vi "sample rack.vi"(0 "Sample Tray":T2, 1 "vial status":enum16{"Empty", "Filling", "Full"}[](array[ring]), 2 "colors":u32[](array[colorbox])=[61185, 16383786, 2621695], 4 "Gilson ID":i32) -> (3 "scale":dbl[unit], 5 "vial position":T5, 6 "Sample Tray out":T2)   [LabVIEW 2012]
uses:
  point.ctl
  file action.ctl
  vial position.ctl
  toolbar icons/Save calibration.ctl
  toolbar icons/Open calibration.ctl
panel:
  out "Coords":cluster{"Horizontal":i32, "Vertical":i32}
  out "Array":bool[](array[boolean])
  out "vial radius":dbl
  out "vial graph centers":cluster{"x":dbl, "y":dbl}[](array[cluster])
  in  "Open sample tray":T3
  in  "Save sample tray":T4
  in  "OK Button":bool
  in  "Model 222 range":T1={"x"=0.39299999999999996, "y"=0.244}
  out "sample tray":picture
  # "Click on vial to move sample changer to that position"
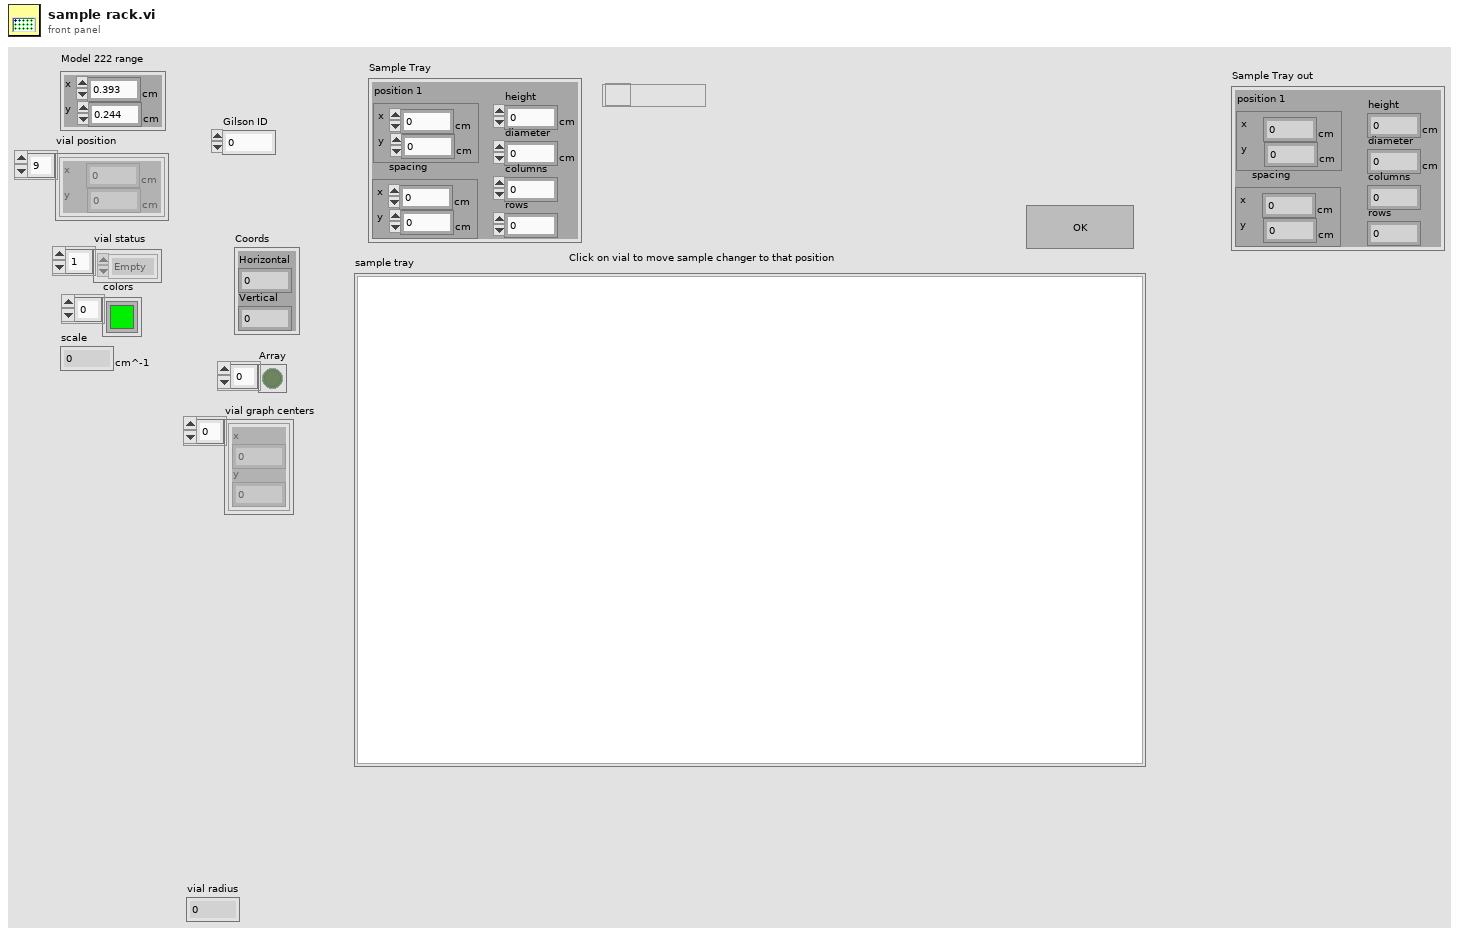
[diagram p1: front panel]
types:
  T1 = typedef "point.ctl" = cluster{"x":dbl[unit], "y":dbl[unit]}
  T2 = cluster{"diameter":dbl[unit], "height":dbl[unit], "columns":u16, "rows":u16, "position 1":T1, "spacing":T1}
  T3 = typedef "Open calibration.ctl" = bool
  T4 = typedef "Save calibration.ctl" = bool
  T5 = typedef "vial position.ctl" = T1[]
  T6 = cluster{"Width":u16, "Style":enum32{"Solid", "Dash", "Dot", "DashDot", "DashDotDot"}}
  T7 = typedef "file action.ctl" = enum16{"Save", "Open"}
  T8 = typedef "LVBoundsTypeDef.ctl" = cluster{"Width":u32, "Height":u32}
  T9 = typedef "LVMouseTypeDef.ctl" = cluster{"Mouse Position":cluster{"X":i32, "Y":i32}, "Mouse Modifiers":cluster{"Button Down":bool, "Shift Mod":bool, "Menu Mod":bool, "Option Mod":bool}}
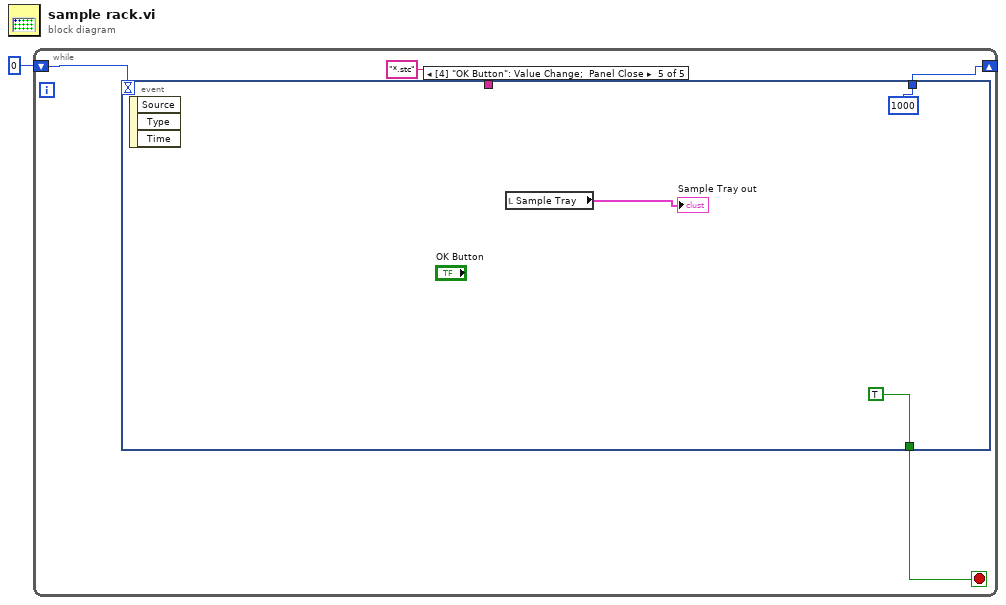
[diagram p0: block diagram]
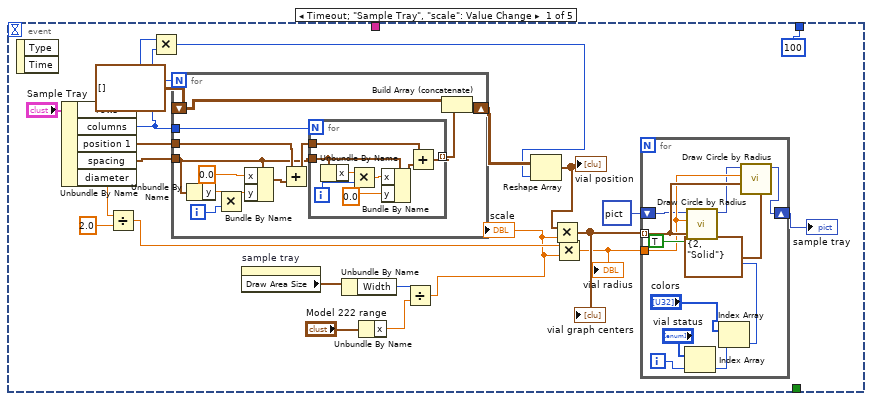
[diagram p2: hidden frame]
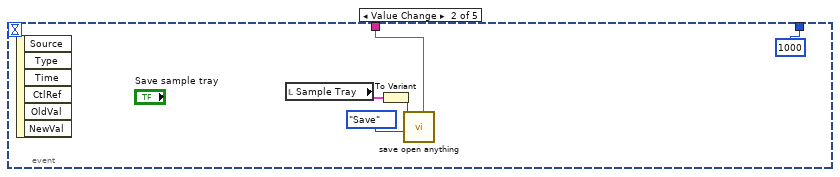
[diagram p3: hidden frame]
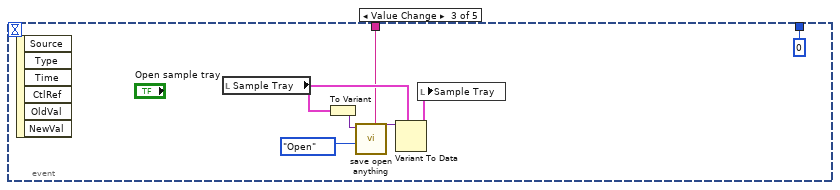
[diagram p4: hidden frame]
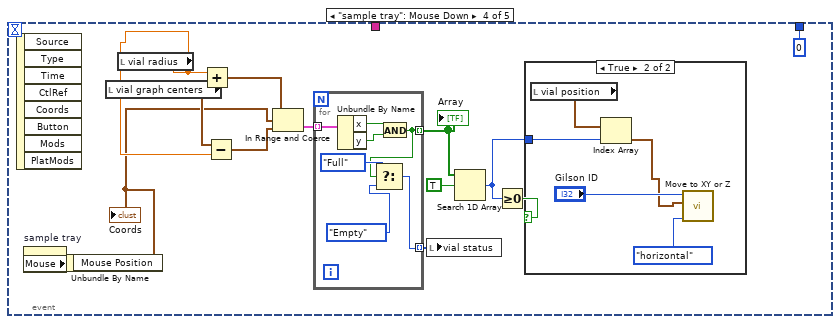
[diagram p5: hidden frame]
diagram:
  n1 = while {
    shift-right: [w3] -> _
    shift-left: 0 -> [w2]
    stop <- w5 stop-if-true
    n2 = event shown="[4] \"OK Button\": Value Change;  Panel Close" {
      selector: _ -> [_ _ _ _ _]
      dyn-events: _ -> [_ _ _ _ _]
      timeout: w2 -> [_ _ _ _ _]
      tunnel: [_ _ _ _ TRUE] -> w5
      tunnel: "*.stc" ("pattern") -> [_ w61 w66 _ _]
      tunnel: [100 1000 0 0 1000] -> w3
      event Timeout; "Sample Tray", "scale": Value Change {
        n3 = event-data() -> ()  [unwired: 1 in, 2 out]
        n4 = Unbundle By Name("Sample Tray") -> ("rows"=w23:u16, "columns"=w22:u16, "position 1"=w26:T1, "spacing"=w25:T1, "diameter"=w20:dbl[unit])
        n5 = Divide(x=w20, y=2.0) -> (x/y=w14:dbl[unit])
        n6 = Multiply(x=w23, y=w22) -> (x*y=w21:u16)
        n7 = for {
          N: w23 -> [_]
          tunnel: w22 -> [w51]
          tunnel: w26 -> [w43]
          tunnel: w25 -> [w40]
          shift-right: [w50] -> w24
          shift-left: T1[][] [] -> [w49]
          i -> [w47]
          n8 = Unbundle By Name(w40) -> ("y"=w46:dbl[unit])
          n9 = Multiply(x=w46, y=w47) -> (x*y=w45:dbl[unit])
          n10 = Bundle By Name(cluster=w40, "x"=dbl[unit] 0.0, "y"=w45) -> (w44:T1)
          n11 = Add(x=w43, y=w44) -> (x+y=w42:T1)
          n12 = for {
            N: w51 -> [_]
            tunnel: w42 -> [w57]
            tunnel: w40 -> [w54]
            tunnel: [w55] -> w48 mode=indexing
            i -> [w53]
            n13 = Unbundle By Name(w54) -> ("x"=w59:dbl[unit])
            n14 = Multiply(x=w59, y=w53) -> (x*y=w58:dbl[unit])
            n15 = Bundle By Name(cluster=w54, "x"=w58, "y"=dbl[unit] 0.0 ("x")) -> (w56:T1)
            n16 = Add(x=w57, y=w56) -> (x+y=w55:T1)
          }
          n17 = Build Array (concatenate)(w49, w48) -> (w50:T1[][])
        }
        n18 = property on="sample tray" class="Pict"() -> ("Draw Area Size"=w11:T8)  [unwired: 2 in, 2 out]
        n19 = Unbundle By Name(w11) -> ("Width"=w8:u32)
        n20 = Unbundle By Name("Model 222 range") -> ("x"=w7:dbl[unit])
        n21 = Divide(x=w8, y=w7) -> (x/y=w9:dbl[unit])
        "scale" <- w9
        n22 = Reshape Array(w24, w21) -> (w16:T1[])
        "vial position" <- w16
        n23 = Multiply(x=w16, y=w9) -> (x*y=w15:cluster{"x":dbl, "y":dbl}[])
        "vial graph centers" <- w15
        n24 = Multiply(x=w14, y=w9) -> (x*y=w13:dbl)
        "vial radius" <- w13
        n25 = for {
          tunnel: w15 -> [w36] mode=indexing
          tunnel: w13 -> [w35]
          shift-right: [w32] -> w18
          shift-left: picture data[5B] ("new picture") -> [w34]
          i -> [w29]
          n26 = Index Array(array="vial status", index=w29) -> (element=w28:enum16{"Empty", "Filling", "Full"})
          n27 = Index Array(array="colors", index=w28) -> (element=w37:u32)
          n28 = call <vilib>:"Draw Circle by Radius.vi"("color(black)"=w37, "fill?(F)"=TRUE, "pixel center"=w36, "radius"=w35, "picture"=w34) -> ("new picture"=w33:picture)  [unwired: 6 in]
          n29 = call <vilib>:"Draw Circle by Radius.vi"("pen"=T6 {"Width"=2, "Style"=enum."Solid"}, "pixel center"=w36, "radius"=w35, "picture"=w33) -> ("new picture"=w32:picture)  [unwired: 7 in]
        }
        "sample tray" <- w18
      }
      event Value Change {
        n30 = event-data() -> ()  [unwired: 1 in, 6 out]
        n31 = local read "Sample Tray"() -> (w62:T2)
        n32 = To Variant(anything=w62) -> (Variant=w63:variant)
        n33 = call "save open anything.vi"("Variant"=w63, "Action"=file_action."Save", "pattern"=w61) -> ()  [unwired: 4 in, 4 out]
      }
      event Value Change {
        n34 = event-data() -> ()  [unwired: 1 in, 6 out]
        n35 = local read "Sample Tray"() -> (w67:T2)
        n36 = To Variant(anything=w67) -> (Variant=w69:variant)
        n37 = call "save open anything.vi"("Variant"=w69, "Action"=file_action."Open", "pattern"=w66) -> ("Variant out"=w70:variant)  [unwired: 4 in, 3 out]
        n38 = Variant To Data(type=w67, Variant=w70) -> (data=w68:T2)  [unwired: 1 in, 1 out]
        n39 = local write "Sample Tray"(w68) -> ()
      }
      event "sample tray": Mouse Down {
        n40 = event-data() -> ()  [unwired: 1 in, 8 out]
        n41 = property on="sample tray" class="Pict"() -> ("Mouse"=w75:T9)  [unwired: 2 in, 2 out]
        n42 = Unbundle By Name(w75) -> ("Mouse Position"=w74:cluster{"X":i32, "Y":i32})
        "Coords" <- w74
        n43 = local read "vial graph centers"() -> (w83:cluster{"x":dbl, "y":dbl}[])
        n44 = local read "vial radius"() -> (w82:dbl)
        n45 = Add(x=w82, y=w83) -> (x+y=w84:cluster{"x":dbl, "y":dbl}[])
        n46 = Subtract(x=w83, y=w82) -> (x-y=w81:cluster{"x":dbl, "y":dbl}[])
        n47 = In Range and Coerce(upper limit=w84, x=w74, lower limit=w81) -> (In Range?=w80:cluster{"x":bool, "y":bool}[])  [unwired: 1 out]
        n48 = for {
          tunnel: w80 -> [w96] mode=indexing
          tunnel: [w90] -> w79 mode=indexing
          tunnel: [w91] -> w72 mode=indexing
          n49 = Unbundle By Name(w96) -> ("x"=w95:bool, "y"=w94:bool)
          n50 = And(x=w95, y=w94) -> (x .and. y?=w90:bool)
          n51 = Select(t=enum16{"Empty", "Filling", "Full"}."Full" ("sample status"), s=w90, f=enum16{"Empty", "Filling", "Full"}."Empty" ("sample status")) -> (s? t:f=w91:enum16{"Empty", "Filling", "Full"})
        }
        "Array" <- w79
        n52 = local write "vial status"(w72) -> ()
        n53 = Search 1D Array(1D array=w79, element=TRUE) -> (index of element=w76:i32)  [unwired: 1 in]
        n54 = Greater Or Equal To 0?(x=w76) -> (x >= 0?=w77:bool)
        n55 = case shown="True" w77 {
          tunnel: w76 -> [_ w86]
          frame False {
          }
          frame True {
            n56 = local read "vial position"() -> (w87:T5)
            n57 = Index Array(array=w87, index=w86) -> (element=w85:T1)
            n58 = call "Move to XY or Z.vi"("move type"=enum16{"horizontal", "vertical"}."horizontal", "position 1"=w85, "ID"="Gilson ID") -> ()  [unwired: 7 in, 2 out]
          }
        }
      }
      event "OK Button": Value Change; Panel Close {
        n59 = event-data() -> ()  [unwired: 1 in, 3 out]
        n60 = local read "Sample Tray"() -> (→"Sample Tray out":T2)
      }
    }
  }
